vi "niDTS BT BDR Tx Test Close.vi"(0 "Dummy Test Handle out":T1, 11 "error in (no error)":errorcluster) -> (15 "error out":errorcluster)   [LabVIEW 2014, in "niDTS BT.lvlib"]
uses:
  niDTS BT.lvlib
  Tx Test/Includes/niDTS BT Tx Test INC Handle.ctl
  Tx Test/Objects/BASE_class/niDTS BT Tx Test.lvclass
  Framework/Session/Includes/niDTS Session INC Force Destroy.ctl
  Framework/niDTS Framework.lvlib
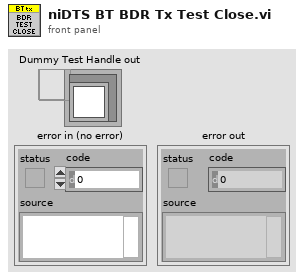
[diagram p1: front panel]
types:
  T1 = typedef "niDTS BT.lvlib/niDTS BT Tx Test INC Handle.ctl" = refnum<data-value>
  T2 = typedef "niDTS Framework.lvlib/niDTS Session INC Force Destroy.ctl" = bool
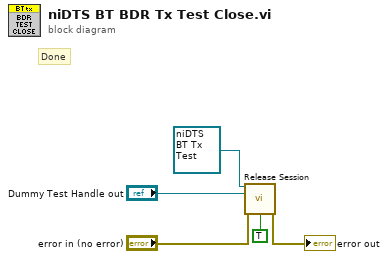
[diagram p0: block diagram]
diagram:
  # "Done"
  n1 = call-dynamic "Release Session.vi"("OBJ - Session in"=refnum<class "niDTS BT Tx Test.lvclass"> refnum ("Dummy Test.lvlib:Dummy Test.lvclass"), "Session Handle in"="Dummy Test Handle out", "error in (no error)"="error in (no error)", "Force Destroy? (F)"=T2 TRUE) -> ("error out"=→"error out":errorcluster)  [unwired: 10 in, 1 out]
